vi "Tektronix Init_n_Config.vi"(5 "End Point":i32, 7 "Start Point":i32, 8 "error in (no error)":errorcluster, 9 "Waveform Width":u8(knob)=1 min=1 max=2 step=1 scale=0.0..2.0, 10 "# Average":u8(ring)=4 items=["128"=128, "64"=64, "16"=16, "4"=4], 11 "Tektronix (0::20:)":refnum<visa-resource-name>) -> (0 "error out":errorcluster, 1 "Waveform Parameters":string, 2 "Acquire Parameters":string, 3 "VISA resource name out":refnum<visa-resource-name>, 4 "concatenated string":string)   [LabVIEW 2018]
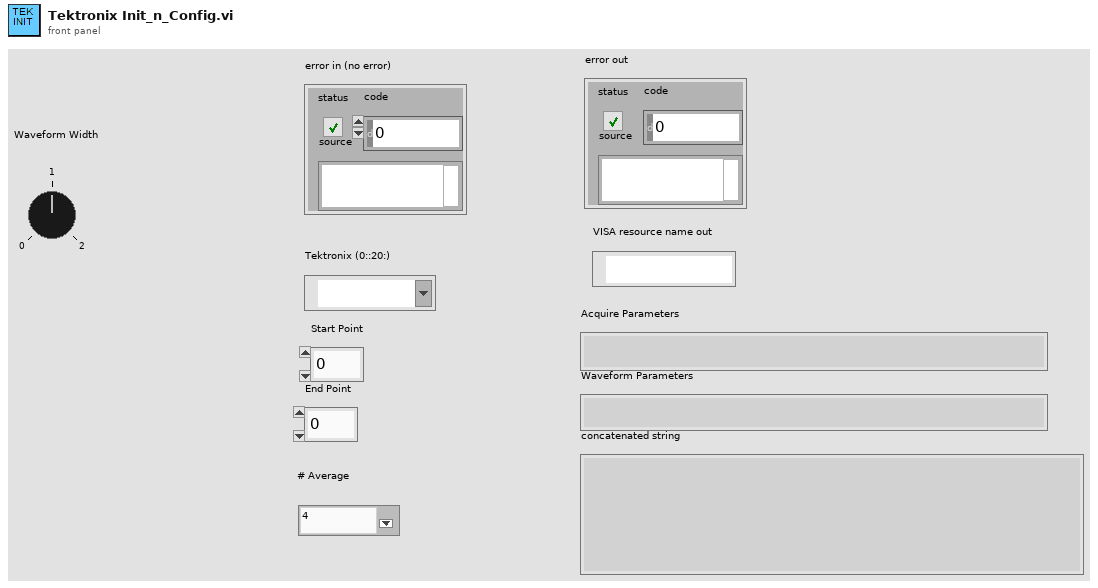
[diagram p1: front panel]
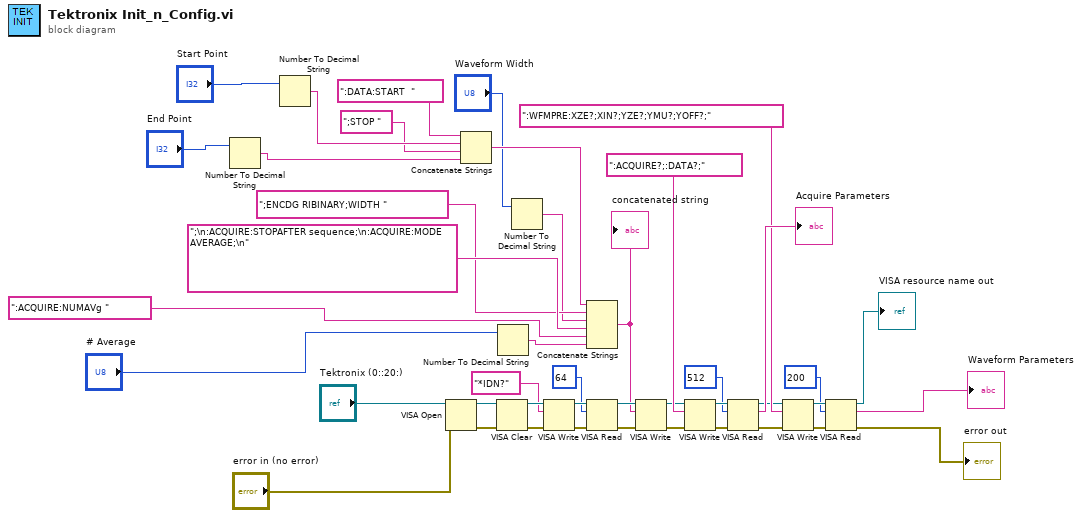
[diagram p0: block diagram]
diagram:
  n1 = Number To Decimal String(number="End Point") -> (decimal integer string=w9:string)  [unwired: 1 in]
  n2 = Number To Decimal String(number="Start Point") -> (decimal integer string=w11:string)  [unwired: 1 in]
  n3 = VISA Open(error in (no error)="error in (no error)", VISA resource name="Tektronix (0::20:)") -> (VISA resource name=w41:refnum<visa-resource-name>, error out=w42:errorcluster)  [unwired: 3 in]
  n4 = Concatenate Strings(":DATA:START  " ("string"), w11, ";STOP " ("string"), w9) -> (w4:string)
  n5 = VISA Clear(VISA resource name=w41, error in (no error)=w42) -> (VISA resource name out=w39:refnum<visa-resource-name>, error out=w40:errorcluster)
  n6 = Number To Decimal String(number="# Average") -> (decimal integer string=w16:string)  [unwired: 1 in]
  n7 = Number To Decimal String(number="Waveform Width") -> (decimal integer string=w1:string)  [unwired: 1 in]
  n8 = VISA Write(VISA resource name=w39, write buffer="*IDN?", error in (no error)=w40) -> (VISA resource name out=w37:refnum<visa-resource-name>, error out=w36:errorcluster)  [unwired: 1 out]
  n9 = Concatenate Strings(w4, ";ENCDG RIBINARY;WIDTH " ("write buffer"), w1, ";\n:ACQUIRE:STOPAFTER sequence;\n:ACQUIRE:MODE AVERAGE;\n" ("write buffer"), ":ACQUIRE:NUMAVg " ("string"), w16) -> (w18:string)
  "concatenated string" <- w18
  n10 = VISA Read(VISA resource name=w37, byte count=u32 64, error in (no error)=w36) -> (VISA resource name out=w30:refnum<visa-resource-name>, error out=w29:errorcluster)  [unwired: 2 out]
  n11 = VISA Write(VISA resource name=w30, write buffer=w18, error in (no error)=w29) -> (VISA resource name out=w23:refnum<visa-resource-name>, error out=w28:errorcluster)  [unwired: 1 out]
  n12 = VISA Write(VISA resource name=w23, write buffer=":ACQUIRE?;:DATA?;", error in (no error)=w28) -> (VISA resource name out=w34:refnum<visa-resource-name>, error out=w33:errorcluster)  [unwired: 1 out]
  n13 = VISA Read(VISA resource name=w34, byte count=u32 512, error in (no error)=w33) -> (VISA resource name out=w5:refnum<visa-resource-name>, read buffer=→"Acquire Parameters":string, error out=w27:errorcluster)  [unwired: 1 out]
  n14 = VISA Write(VISA resource name=w5, write buffer=":WFMPRE:XZE?;XIN?;YZE?;YMU?;YOFF?;", error in (no error)=w27) -> (VISA resource name out=w24:refnum<visa-resource-name>, error out=w26:errorcluster)  [unwired: 1 out]
  n15 = VISA Read(VISA resource name=w24, byte count=u32 200, error in (no error)=w26) -> (VISA resource name out=→"VISA resource name out":refnum<visa-resource-name>, read buffer=→"Waveform Parameters":string, error out=→"error out":errorcluster)  [unwired: 1 out]
